vi "CTRE_Phoenix_CANdle_StrobeAnimation.vi"(0 "CTRE_CANdle_DeviceRef":T2, 5 "Speed":dbl=1.0 min=0.0 max=1.0 step=0.0001, 7 "Num LEDs":i32=-1, 9 "LED Color":T1, 11 "error in":errorcluster) -> (4 "CTRE_CANdle_DeviceRef":T2, 15 "error out":errorcluster)   [LabVIEW 2020]
doc: "Animation that strobes the LEDs a specified color\n\n<b>Speed</b> adjust the speed at which the animation runs. Valid values range from 0 to 1 where 1 is the fastest animation speed.\n\n<b>Num LEDs</b> defines the total number of LEDs to use for the animation.\n\n<b>LED Color</b> is the RGB(W) value of the color to illuminate.s"
uses:
  <vilib>/Rock Robotics/WPI/ThirdParty/Phoenix-LabVIEW/CANdle/Controls/CTRE_Phoenix_CANdle_DeviceRef.ctl
  <vilib>/Rock Robotics/WPI/ThirdParty/Phoenix-LabVIEW/CANdle/Controls/CTRE_Phoenix_CANdle_LEDColor.ctl
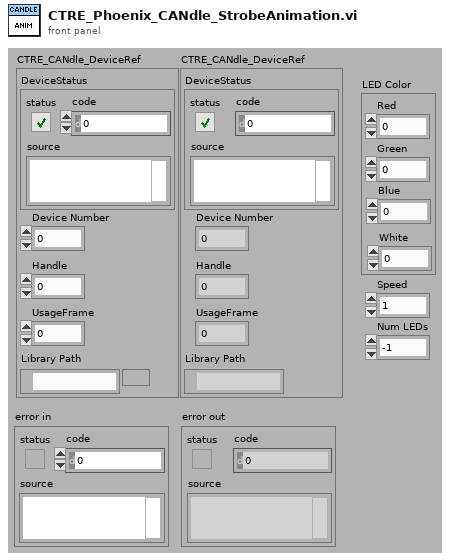
[diagram p1: front panel]
types:
  T1 = typedef "CTRE_Phoenix_CANdle_LEDColor.ctl" = cluster{"Red":u8, "Green":u8, "Blue":u8, "White":u8}
  T2 = typedef "CTRE_Phoenix_CANdle_DeviceRef.ctl" = cluster{"DeviceStatus":errorcluster, "Device Number":u8, "Handle":u64, "UsageFrame":u32, "Library Path":path}
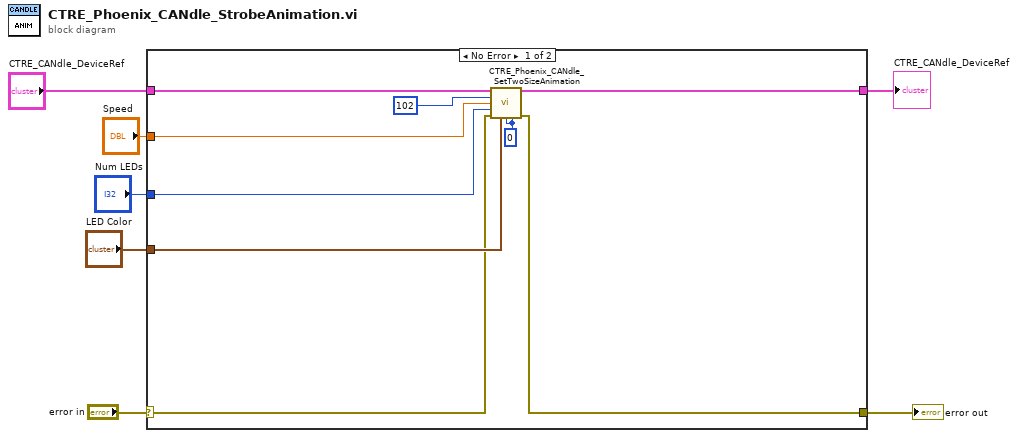
[diagram p0: block diagram]
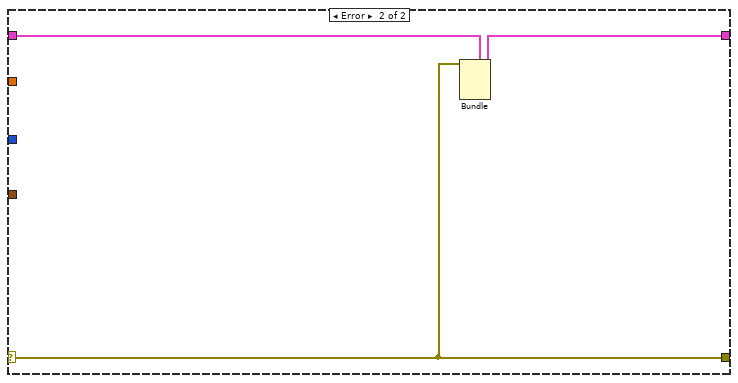
[diagram p2: hidden frame]
diagram:
  n1 = case shown="No Error" "error in" {
    selector: "error in" -> [w10 w18]
    tunnel: "CTRE_CANdle_DeviceRef" -> [w16 w19]
    tunnel: [w9 w18] -> w7
    tunnel: [w15 w17] -> w4
    tunnel: "LED Color" -> [w14 _]
    tunnel: "Speed" -> [w12 _]
    tunnel: "Num LEDs" -> [w11 _]
    frame No Error {
      w8 = 0 ("size")
      n2 = call <vilib>:"CTRE_Phoenix_CANdle_SetTwoSizeAnimation.vi"("CTRE_CANdle_DeviceRef"=w16, "idx"=102, "speed"=w12, "numLED"=w11, "error in"=w10, "LED Color"=w14, "direction"=w8, "size"=w8) -> ("CTRE_CANdle_DeviceRef"=w15:T2, "error out"=w9:errorcluster)  [unwired: 6 in]
    }
    frame Error {
      n3 = Bundle(cluster=w19, "DeviceStatus"=w18) -> (w17:T2)  [unwired: 4 in]
    }
  }
  "error out" <- w7
  "CTRE_CANdle_DeviceRef" <- w4
